vi "channeldata_bigendian.vi"() -> ()   [LabVIEW 2019]
panel:
  out "Error Out":errorcluster
  in  "TDMS File":path=path "C:/Python/projects/nitdms/tests/tdms_files/channeldata_bigendian.tdms"
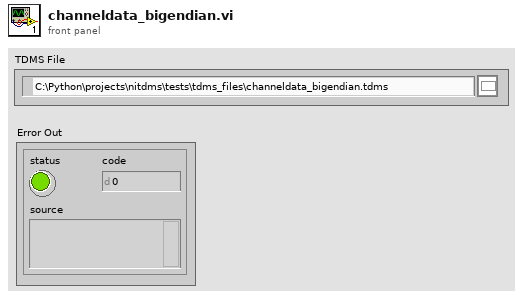
[diagram p1: front panel]
types:
  T1 = enum16{"big-endian, network order", "native, host order", "little-endian"}
  T2 = enum16{"open", "open or create", "create or replace", "create", "open (read-only)"}
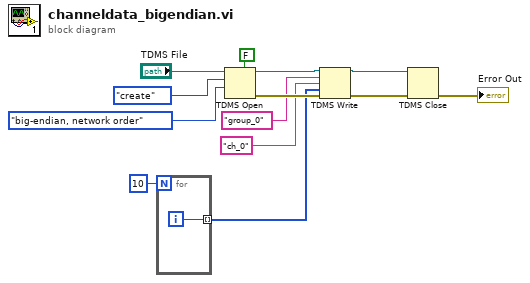
[diagram p0: block diagram]
diagram:
  n1 = for {
    N: 10 -> [_]
    tunnel: [w14] -> w2 mode=indexing
    i -> [w14]
  }
  n2 = TDMS Open(5:FALSE ("create index file? (T)"), 9:T1."big-endian, network order" ("byte order (2:little-endian)"), 10:T2."create" ("operation (0:open)"), 11:"TDMS File") -> (0:w9:errorcluster, 3:w8:refnum<k34>)  [unwired: 3 in]
  n3 = TDMS Write(0:w8, 5:"group_0", 7:"ch_0", 9:w2, 11:w9) -> (4:w6:refnum<k34>, 15:w7:errorcluster)  [unwired: 1 in, 2 out]
  n4 = TDMS Close(8:w7, 11:w6) -> (0:→"Error Out":errorcluster)  [unwired: 1 out]
